vi "T7_Read_UINT16_Register.vi"(9 "FirstChannel":i32, 10 "Remote Port":u16=502, 11 "Remote IP Address":string="192.168.126.148") -> (2 "LastValue":dbl, 3 "Array":dbl[](array[numeric]))   [LabVIEW 2014]
uses:
  Serial Link Layer/NI_Modbus_Cleaned/NI Modbus121Clean.llb/MB Ethernet Master Query Read Input Registers (poly).vi
panel:
  in  "Num Registers to read":i32=2
  out "Read UINT16":u16
  out "Raw Data Read":u16[](array[numeric])
  # "MB Ethernet Example Master.vi\n\nInstructions\n1.Use Kipling to find your devices IP address & modify the\n\"Remote IP Addres\"\n2. Run this VI\n3. Change value of \"UINT16 to Write\" & press \"Write Data\""
  # "TCP Parameters"
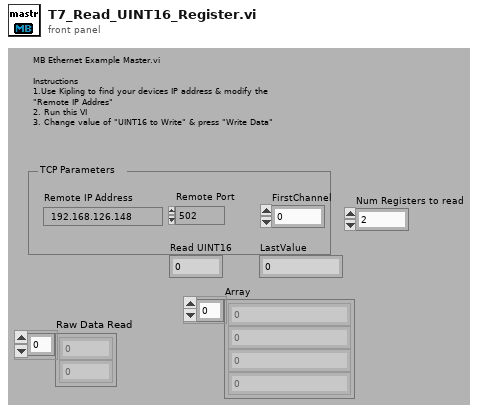
[diagram p1: front panel]
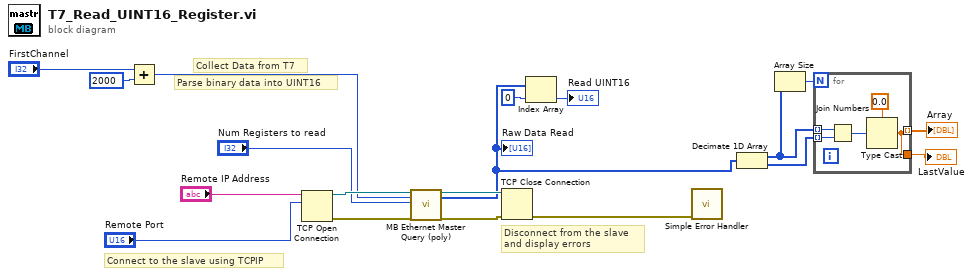
[diagram p0: block diagram]
diagram:
  # "Parse binary data into UINT16"
  # "Collect Data from T7"
  # "Disconnect from the slave\nand display errors"
  # "Connect to the slave using TCPIP"
  n1 = Add(x="FirstChannel", y=2000) -> (x+y=w8:i32)
  n2 = TCP Open Connection(address="Remote IP Address", remote port or service name="Remote Port") -> (connection ID=w17:refnum<k5>, error out=w16:errorcluster)  [unwired: 3 in]
  n3 = call-poly "MB Ethernet Master Query (poly).vi"("TCP Connection Refnum in"=w17, "Starting Address"=w8, "Quantity"="Num Registers to read", "error in"=w16) -> ("TCP Connection Refnum (dup)"=w13:refnum<k5>, "Input Registers"=w1:u16[], "error out"=w14:errorcluster)  [unwired: 12 in, 1 out]
  "Raw Data Read" <- w1
  n4 = TCP Close Connection(connection ID=w13, error in (no error)=w14) -> (error out=w15:errorcluster)  [unwired: 2 out]
  n5 = Index Array(array=w1, index=0) -> (element=→"Read UINT16":u16)
  n6 = call <vilib>:"Simple Error Handler.vi"("error in (no error)"=w15) -> ()  [unwired: 1 in, 8 out]
  n7 = Decimate 1D Array(w1) -> (w3:u16[], w4:u16[])
  n8 = Array Size(array=w3) -> (size(s)=w2:i32)
  n9 = for {
    N: w2 -> [_]
    tunnel: w3 -> [w23] mode=indexing
    tunnel: w4 -> [w24] mode=indexing
    tunnel: [w20] -> w5 mode=indexing
    tunnel: [w20] -> w6
    n10 = Join Numbers(hi=w23, lo=w24) -> ((hi.lo)=w22:u32)
    n11 = Type Cast(type=sgl 0.0, x=w22) -> (*(type *) &x=w20:sgl)
  }
  "Array" <- w5
  "LastValue" <- w6
